vi "ExcelOpenFile.vi"(8 "error in (no error)":errorcluster, 10 "file":string) -> (0 "error out":errorcluster)   [LabVIEW 2018]
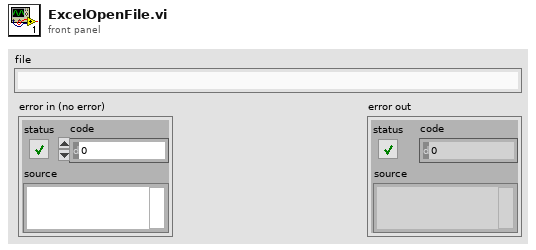
[diagram p1: front panel]
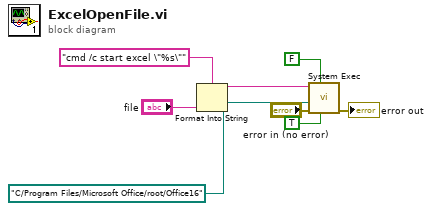
[diagram p0: block diagram]
diagram:
  n1 = Format Into String(format string="cmd /c start excel \"%s\"", "file") -> (resulting string=w6:string)  [unwired: 2 in, 1 out]
  n2 = call <vilib>:"System Exec.vi"("run minimized? (F)"=TRUE, "wait until completion? (T)"=FALSE, "error in (no error)"="error in (no error)", "working directory"=path "C:/Program Files/Microsoft Office/root/Office16", "command line"=w6) -> ("error out"=→"error out":errorcluster)  [unwired: 3 in, 3 out]
